vi "15_DC Motor_PID.vi"() -> ()   [LabVIEW 2018]
uses:
  <userlib>/KNR OS 4.0 LabVIEW Toolkit/Type Definition/Resource.ctl
  <userlib>/KNR OS 4.0 LabVIEW Toolkit/Type Definition/DC Motor Port.ctl
panel:
  in  "Port":T1=4 items=["DS1"=4, "DS2"=5, "DS3"=6, "DS4"=7]
  out "Velocity (cm/sec) Chart":dbl(graph)
  out "Speed (+-100%)":dbl
  in  "Desire Velosity (cm/sec)":dbl(slide) scale=-100.0..100.0
  in  "Kd":dbl(slide)=0.01 scale=0.0..0.02
  in  "Ki":dbl(slide)=0.1 scale=0.0..0.2
  in  "Kp":dbl(slide)=0.5 scale=0.0..1.0
  in  "IP":string(combo)="172.22.11.2"
  in  "Resource":T2=enum."KNRm_DDDD"
  in  "stop":bool
  in  "Enable Motor":bool
  out "Position cm":dbl
  out "Velocity (cm/sec)":dbl
  in  "Reverse?":bool
  in  "Reset":bool
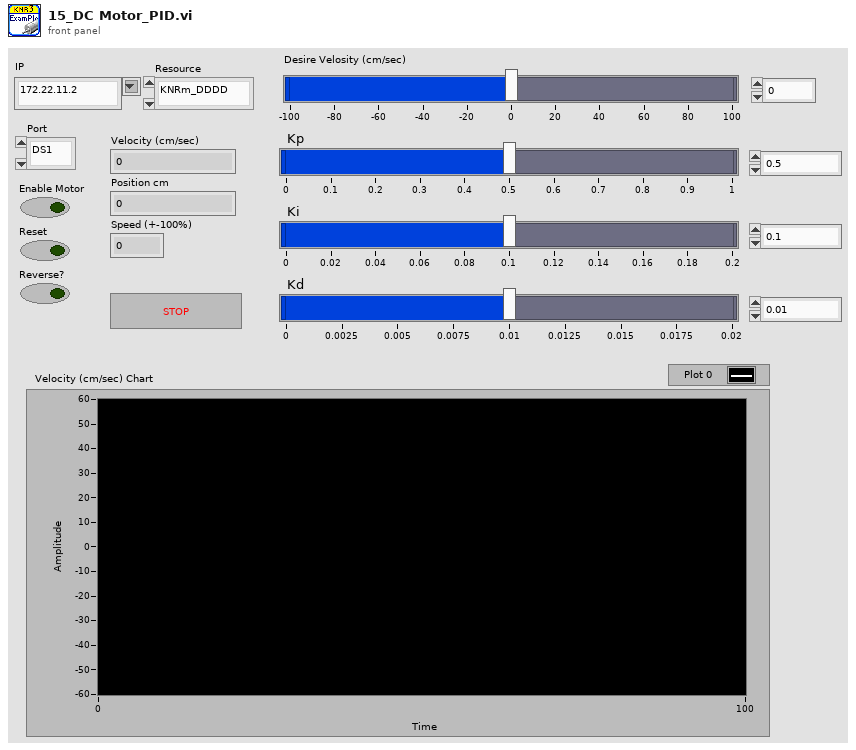
[diagram p1: front panel]
types:
  T1 = typedef "DC Motor Port.ctl" = u16
  T2 = typedef "Resource.ctl" = enum16{"KNRm_DDRC", "KNRm_DDDD", "KNRm_DDDR", "KNRm_DDDC", "KNR", "KNRm_neww"}
  T3 = typedef "KNR3 Reference.ctl" = cluster{"FPGA Session":refnum<class "FPGA Interface Base.lvclass">, "Resource":T2}
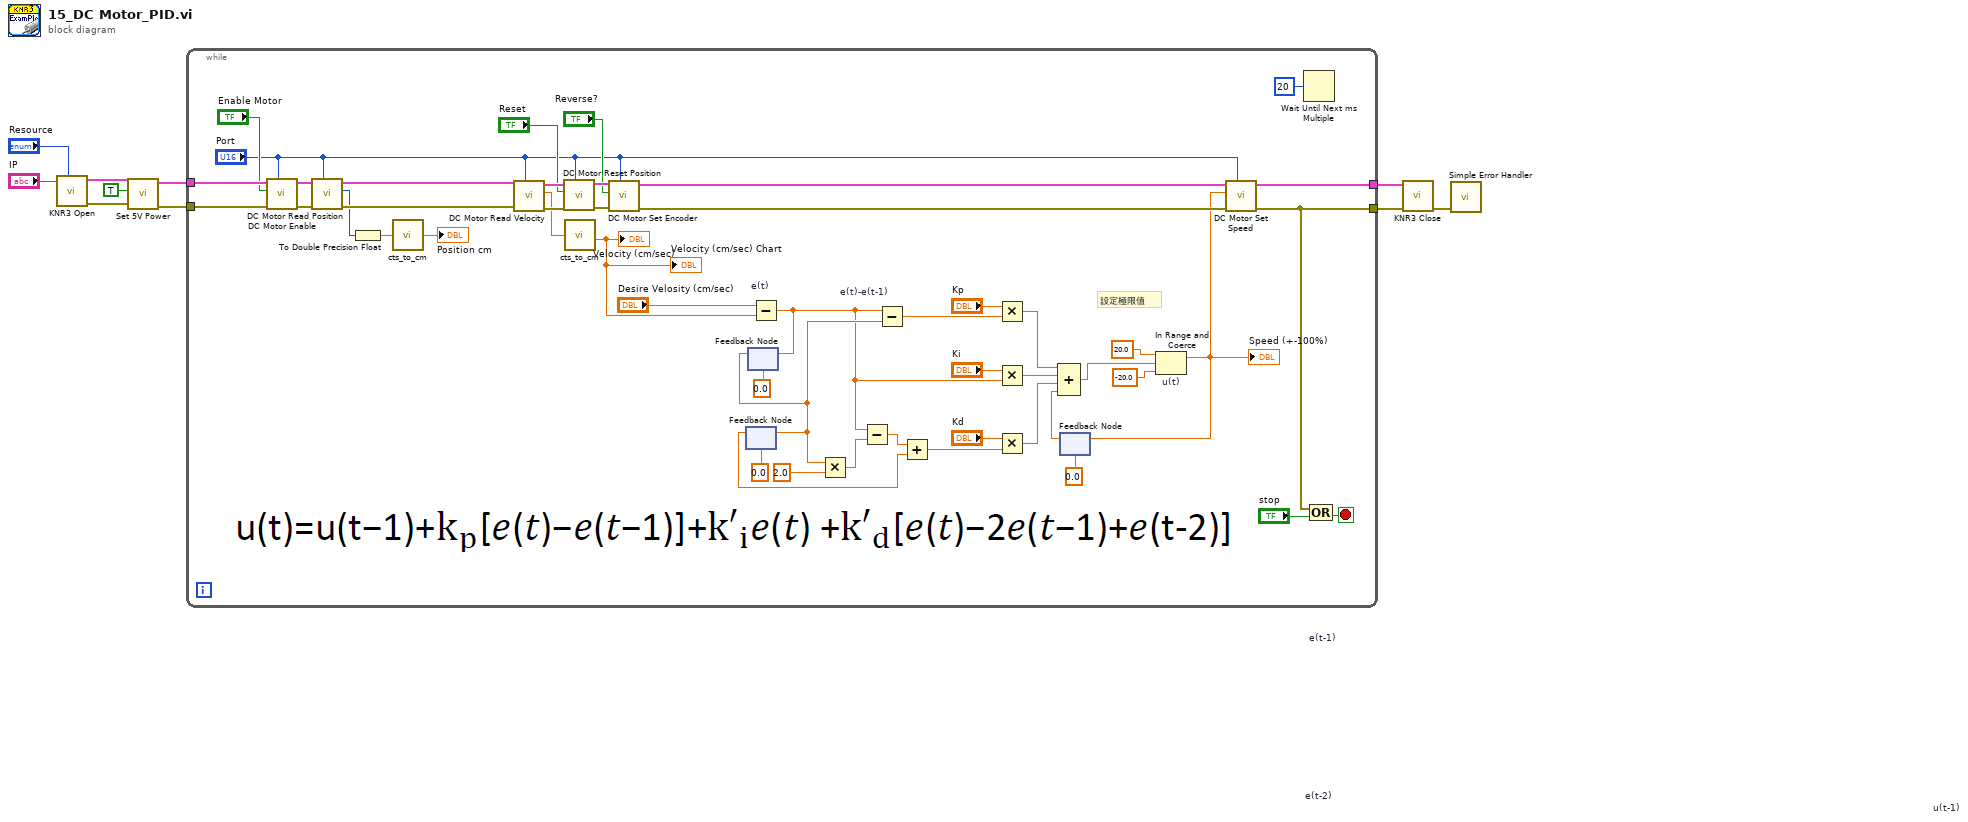
[diagram p0: block diagram]
diagram:
  n1 = call <userlib>:"KNR3 Open.vi"("Resource"="Resource", "IP"="IP") -> ("error out"=w4:errorcluster, "KNR out"=w6:T3)  [unwired: 8 in]
  n2 = call <userlib>:"Set 5V Power.vi"("error in (no error)"=w4, "5V Power(T)"=TRUE ("5V Power"), "KNR in"=w6) -> ("error out"=w8:errorcluster, "KNR out"=w9:T3)  [unwired: 7 in]
  n3 = while {
    tunnel: w9 -> [w59]
    tunnel: w8 -> [w57]
    tunnel: [w13] -> w2
    tunnel: [w12] -> w1
    stop <- w55 stop-if-true
    # "設定極限值"
    n4 = call <userlib>:"DC Motor Enable.vi"("Port (DS1)"="Port", "error in (no error)"=w57, "Enable Motor(F)"="Enable Motor", "KNR in"=w59) -> ("error out"=w18:errorcluster, "KNR out"=w19:T3)  [unwired: 6 in]
    n5 = call <userlib>:"DC Motor Read Position.vi"("Port (DS1)"="Port", "error in (no error)"=w18, "KNR in"=w19) -> ("error out"=w52:errorcluster, "Position"=w43:i32, "KNR out"=w53:T3)  [unwired: 6 in]
    n6 = To Double Precision Float(number=w43) -> (double precision float=w42:dbl)
    n7 = call "cts_to_cm.vi"("cts"=w42) -> ("cm"=→"Position cm":dbl)
    n8 = call <userlib>:"DC Motor Read Velocity.vi"("Port (DS1)"="Port", "error in (no error)"=w52, "KNR in"=w53) -> ("error out"=w48:errorcluster, "Velocity (cts/sec)"=w47:dbl, "KNR out"=w51:T3)  [unwired: 6 in]
    n9 = call <userlib>:"DC Motor Reset Position.vi"("Port (DS1)"="Port", "error in (no error)"=w48, "Reset(F)"="Reset", "KNR in"=w51) -> ("error out"=w49:errorcluster, "KNR out"=w50:T3)  [unwired: 6 in]
    n10 = call "cts_to_cm.vi"("cts"=w47) -> ("cm"=w11:dbl)
    "Velocity (cm/sec)" <- w11
    "Velocity (cm/sec) Chart" <- w11
    n11 = call <userlib>:"DC Motor Set Encoder.vi"("Port (DS1)"="Port", "error in (no error)"=w49, "Reverse?(F)"="Reverse?", "KNR in"=w50) -> ("error out"=w16:errorcluster, "KNR out"=w17:T3)  [unwired: 6 in]
    n12 = feedback #1 "e(t-2)"(0.0) -> (w33:dbl)
    n13 = feedback #2 "e(t-1)"(0.0) -> (w24:dbl)
    n14 = feedback-in #1(w24) -> ()
    n15 = Subtract "e(t)"(x="Desire Velosity (cm/sec)", y=w11) -> (x-y=w23:dbl)
    n16 = feedback-in #2(w23) -> ()
    n17 = Multiply(x=w24, y=2.0) -> (x*y=w31:dbl)
    n18 = Subtract(x=w23, y=w31) -> (x-y=w32:dbl)
    n19 = Subtract "e(t)-e(t-1)"(x=w23, y=w24) -> (x-y=w27:dbl)
    n20 = Add(x=w32, y=w33) -> (x+y=w34:dbl)
    n21 = Multiply(x="Kp", y=w27) -> (x*y=w36:dbl)
    n22 = Multiply(x="Ki", y=w23) -> (x*y=w37:dbl)
    n23 = Multiply(x="Kd", y=w34) -> (x*y=w38:dbl)
    n24 = feedback #3 "u(t-1)"(0.0) -> (w39:dbl)
    n25 = Compound Arithmetic op=ADD(w36, w37, w38, w39) -> (w41:dbl)
    n26 = In Range and Coerce "u(t)"(upper limit=20.0, x=w41, lower limit=-20.0 ("y")) -> (coerced(x)=w14:dbl)  [unwired: 1 out]
    "Speed (+-100%)" <- w14
    n27 = feedback-in #3(w14) -> ()
    n28 = call <userlib>:"DC Motor Set Speed.vi"("Port (DS1)"="Port", "error in (no error)"=w16, "Speed (+-100%)"=w14, "KNR in"=w17) -> ("error out"=w12:errorcluster, "KNR out"=w13:T3)  [unwired: 6 in]
    n29 = Wait Until Next ms Multiple(millisecond multiple=u32 20) -> ()  [unwired: 1 out]
    n30 = Compound Arithmetic op=OR(w12, "stop") -> (w55:bool)
  }
  n31 = call <userlib>:"KNR3 Close.vi"("error in (no error)"=w1, "KNR in"=w2) -> ("error out"=w7:errorcluster)  [unwired: 9 in]
  n32 = call <vilib>:"Simple Error Handler.vi"("error in (no error)"=w7) -> ()  [unwired: 4 in, 5 out]
